vi "Charger_Set Ready Status.vi"(5 "Ready":bool=TRUE, 6 "Status Refnum":T1, 7 "error in":errorcluster) -> (0 "error out":errorcluster {"code" format="%.0x"}, 4 "Ready Status":bool)   [LabVIEW 2020]
uses:
  Charger_Status Refnum.ctl
  Drivers/Charger Test Set/Charger_Input Control.ctl
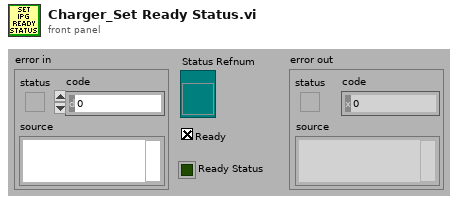
[diagram p1: front panel]
types:
  T1 = typedef "Charger_Status Refnum.ctl" = refnum<vi>
  T2 = typedef "Charger_Input Control.ctl" = cluster{"address":refnum<visa-resource-name>, "position":i32, "setpoint":dbl}
  T3 = cluster{"MICS ID":u32, "VBAT":dbl, "ChargingState":string, "VBAT Slide":dbl, "Status":string, "TemperatureLevel":dbl, "IPG_ReceivedLevel":dbl, "VBAT Target":dbl, "Charger Setpoint":dbl, "Index":i32, "Ready":bool, "Charger Inputs":T2, "MICS Inputs":cluster{"address":refnum<visa-resource-name>, "chan":u16, "ID":u32}}
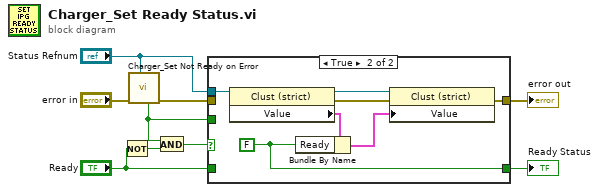
[diagram p0: block diagram]
diagram:
  n1 = Not(x="Ready") -> (.not. x?=w1:bool)
  n2 = call "Charger_Set Not Ready on Error.vi"("Status Refnum"="Status Refnum", "error in"="error in") -> ("error out"=w3:errorcluster, "ready status"=w2:bool)  [unwired: 7 in]
  n3 = And(x=w2, y=w1) -> (x .and. y?=w4:bool)
  n4 = case shown="True" w4 {
    tunnel: "Status Refnum" -> [_ w14]
    tunnel: [w11 w13] -> w8
    tunnel: "Ready" -> [_ _]
    tunnel: [w10 w12] -> w7
    tunnel: w3 -> [w11 _]
    tunnel: w2 -> [w10 _]
    frame False {
    }
    frame True {
      w12 = FALSE ("Ready")
      n5 = property class="Clust (strict)"(reference=w14) -> (reference out=w17:T1, error out=w18:errorcluster, "Value"=w16:T3)  [unwired: 1 in]
      n6 = Bundle By Name(cluster=w16, "Ready"=w12) -> (w15:T3)
      n7 = property class="Clust (strict)"(reference=w17, error in=w18, "Value"=w15) -> (error out=w13:errorcluster)  [unwired: 1 out]
    }
  }
  "error out" <- w8
  "Ready Status" <- w7
